vi "TL27_Display_Fault_Snapshot_Data_Parser rev4.vi"(5 "Input Snao Data":T3) -> (6 "Output Snap Data":T2[](array[typedef]))   [LabVIEW 2016]
uses:
  Get Raw Fault Snapshot Data.ctl
  Control 6.ctl
panel:
  in  "Parser Output Bundle 2":T1
  out "Boolean array":bool[](array[boolean])
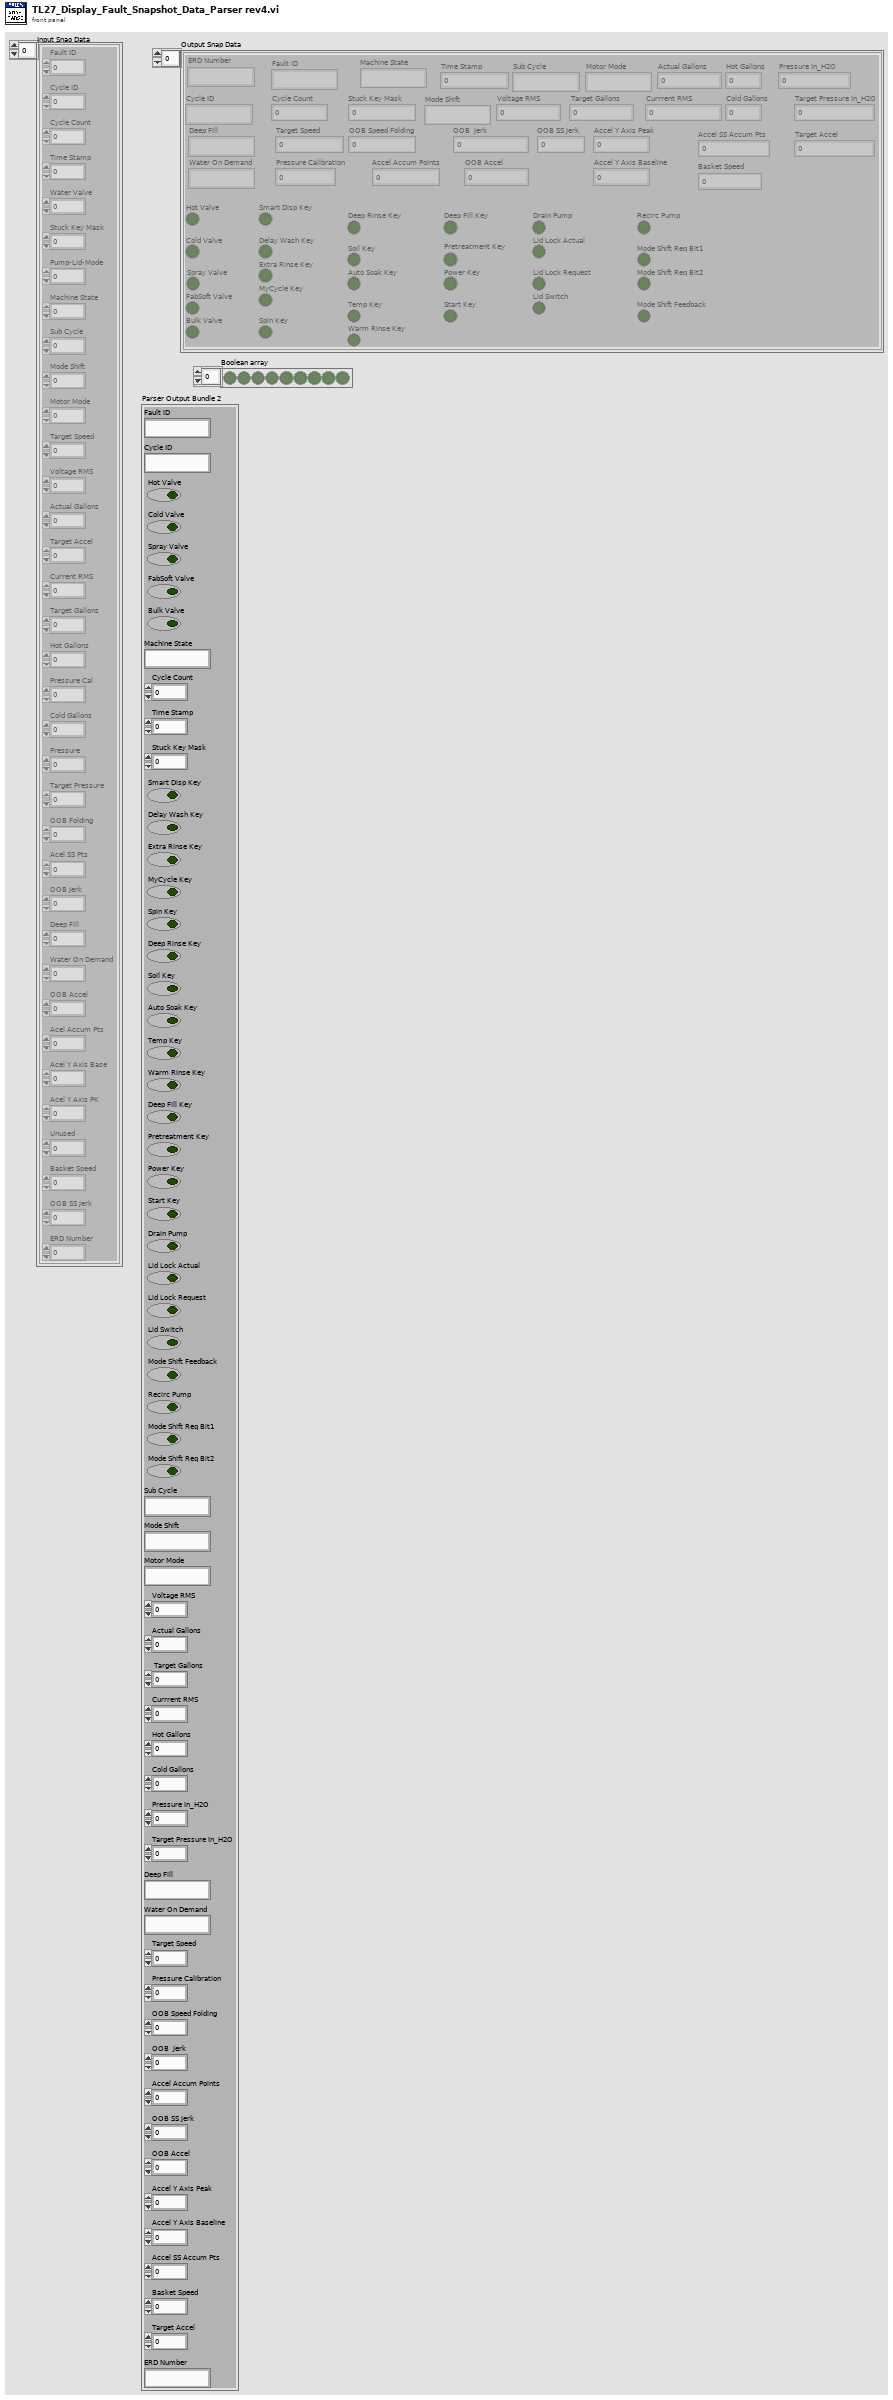
[diagram p1: front panel]
types:
  T1 = cluster{"Fault ID":string, "Cycle ID":string, "Hot Valve":bool, "Cold Valve":bool, "Spray Valve":bool, "FabSoft Valve":bool, "Bulk Valve":bool, "Machine State":string, "Cycle Count":u32, "Time Stamp":u32, "Stuck Key Mask ":u64, "Smart Disp Key":bool, "Delay Wash Key":bool, "Extra Rinse Key":bool, "MyCycle Key":bool, "Spin Key":bool, "Deep Rinse Key":bool, "Soil Key":bool, "Auto Soak Key":bool, "Temp Key":bool, "Warm Rinse Key":bool, "Deep Fill Key":bool, "Pretreatment Key":bool, "Power Key":bool, "Start Key":bool, "Drain Pump":bool, "Lid Lock Actual":bool, "Lid Lock Request":bool, "Lid Switch":bool, "Mode Shift Feedback":bool, "Recirc Pump":bool, "Mode Shift Req Bit1":bool, "Mode Shift Req Bit2":bool, "Sub Cycle":string, "Mode Shift":string, "Motor Mode":string, "Voltage RMS":u16, "Actual Gallons":u16, " Target Gallons":u16, "Currrent RMS":u16, "Hot Gallons":u16, "Cold Gallons":u16, "Pressure In_H2O":u32, "Target Pressure In_H2O":dbl, "Deep Fill":string, "Water On Demand":string, "Target Speed":u16, "Pressure Calibration":u32, "OOB Speed Folding":i32, "OOB  Jerk":i32, "Accel Accum Points":u8, "OOB SS Jerk":i32, "OOB Accel":i32, "Accel Y Axis Peak":i16, "Accel Y Axis Baseline":i16, "Accel SS Accum Pts":u8, "Basket Speed":u16, "Target Accel":u16, "ERD Number":string}
  T2 = typedef "Control 6.ctl" = cluster{"Fault ID":string, "Cycle ID":string, "Hot Valve":bool, "Cold Valve":bool, "Spray Valve":bool, "FabSoft Valve":bool, "Bulk Valve":bool, "Machine State":string, "Cycle Count":u32, "Time Stamp":u32, "Stuck Key Mask ":u64, "Smart Disp Key":bool, "Delay Wash Key":bool, "Extra Rinse Key":bool, "MyCycle Key":bool, "Spin Key":bool, "Deep Rinse Key":bool, "Soil Key":bool, "Auto Soak Key":bool, "Temp Key":bool, "Warm Rinse Key":bool, "Deep Fill Key":bool, "Pretreatment Key":bool, "Power Key":bool, "Start Key":bool, "Drain Pump":bool, "Lid Lock Actual":bool, "Lid Lock Request":bool, "Lid Switch":bool, "Mode Shift Feedback":bool, "Recirc Pump":bool, "Mode Shift Req Bit1":bool, "Mode Shift Req Bit2":bool, "Sub Cycle":string, "Mode Shift":string, "Motor Mode":string, "Voltage RMS":u16, "Actual Gallons":u16, " Target Gallons":u16, "Currrent RMS":u16, "Hot Gallons":u16, "Cold Gallons":u16, "Pressure In_H2O":u32, "Target Pressure In_H2O":dbl, "Deep Fill":string, "Water On Demand":string, "Target Speed":i16, "Pressure Calibration":u32, "OOB Speed Folding":i32, "OOB  Jerk":i32, "Accel Accum Points":u8, "OOB SS Jerk":i32, "OOB Accel":i32, "Accel Y Axis Peak":i16, "Accel Y Axis Baseline":i16, "Accel SS Accum Pts":u8, "Basket Speed":u16, "Target Accel":u16, "ERD Number":string}
  T3 = typedef "Get Raw Fault Snapshot Data.ctl" = cluster{"Fault ID":u16, "Cycle ID":u8, "Cycle Count":u32, "Time Stamp":u32, "Water Valve":u8, "Stuck Key Mask":u64, "Pump-Lid-Mode":u8, "Machine State":u8, "Sub Cycle":u8, "Mode Shift":u8, "Motor Mode":u8, "Target Speed":i16, "Voltage RMS":u16, "Actual Gallons":u16, "Target Accel":u16, "Current RMS":u16, "Target Gallons":u16, "Hot Gallons":u16, "Pressure Cal":u32, "Cold Gallons":u16, "Pressure ":u32, "Target Pressure":u32, "OOB Folding":i32, "Acel SS Pts":u8, "OOB Jerk":i32, "Deep Fill":u8, "Water On Demand":u8, "OOB Accel":i32, "Acel Accum Pts":u8, "Acel Y Axis Base":i16, "Acel Y Axis PK":i16, "Unused":u8, "Basket Speed":u16, "OOB SS Jerk":i32, "ERD Number":u64}[]
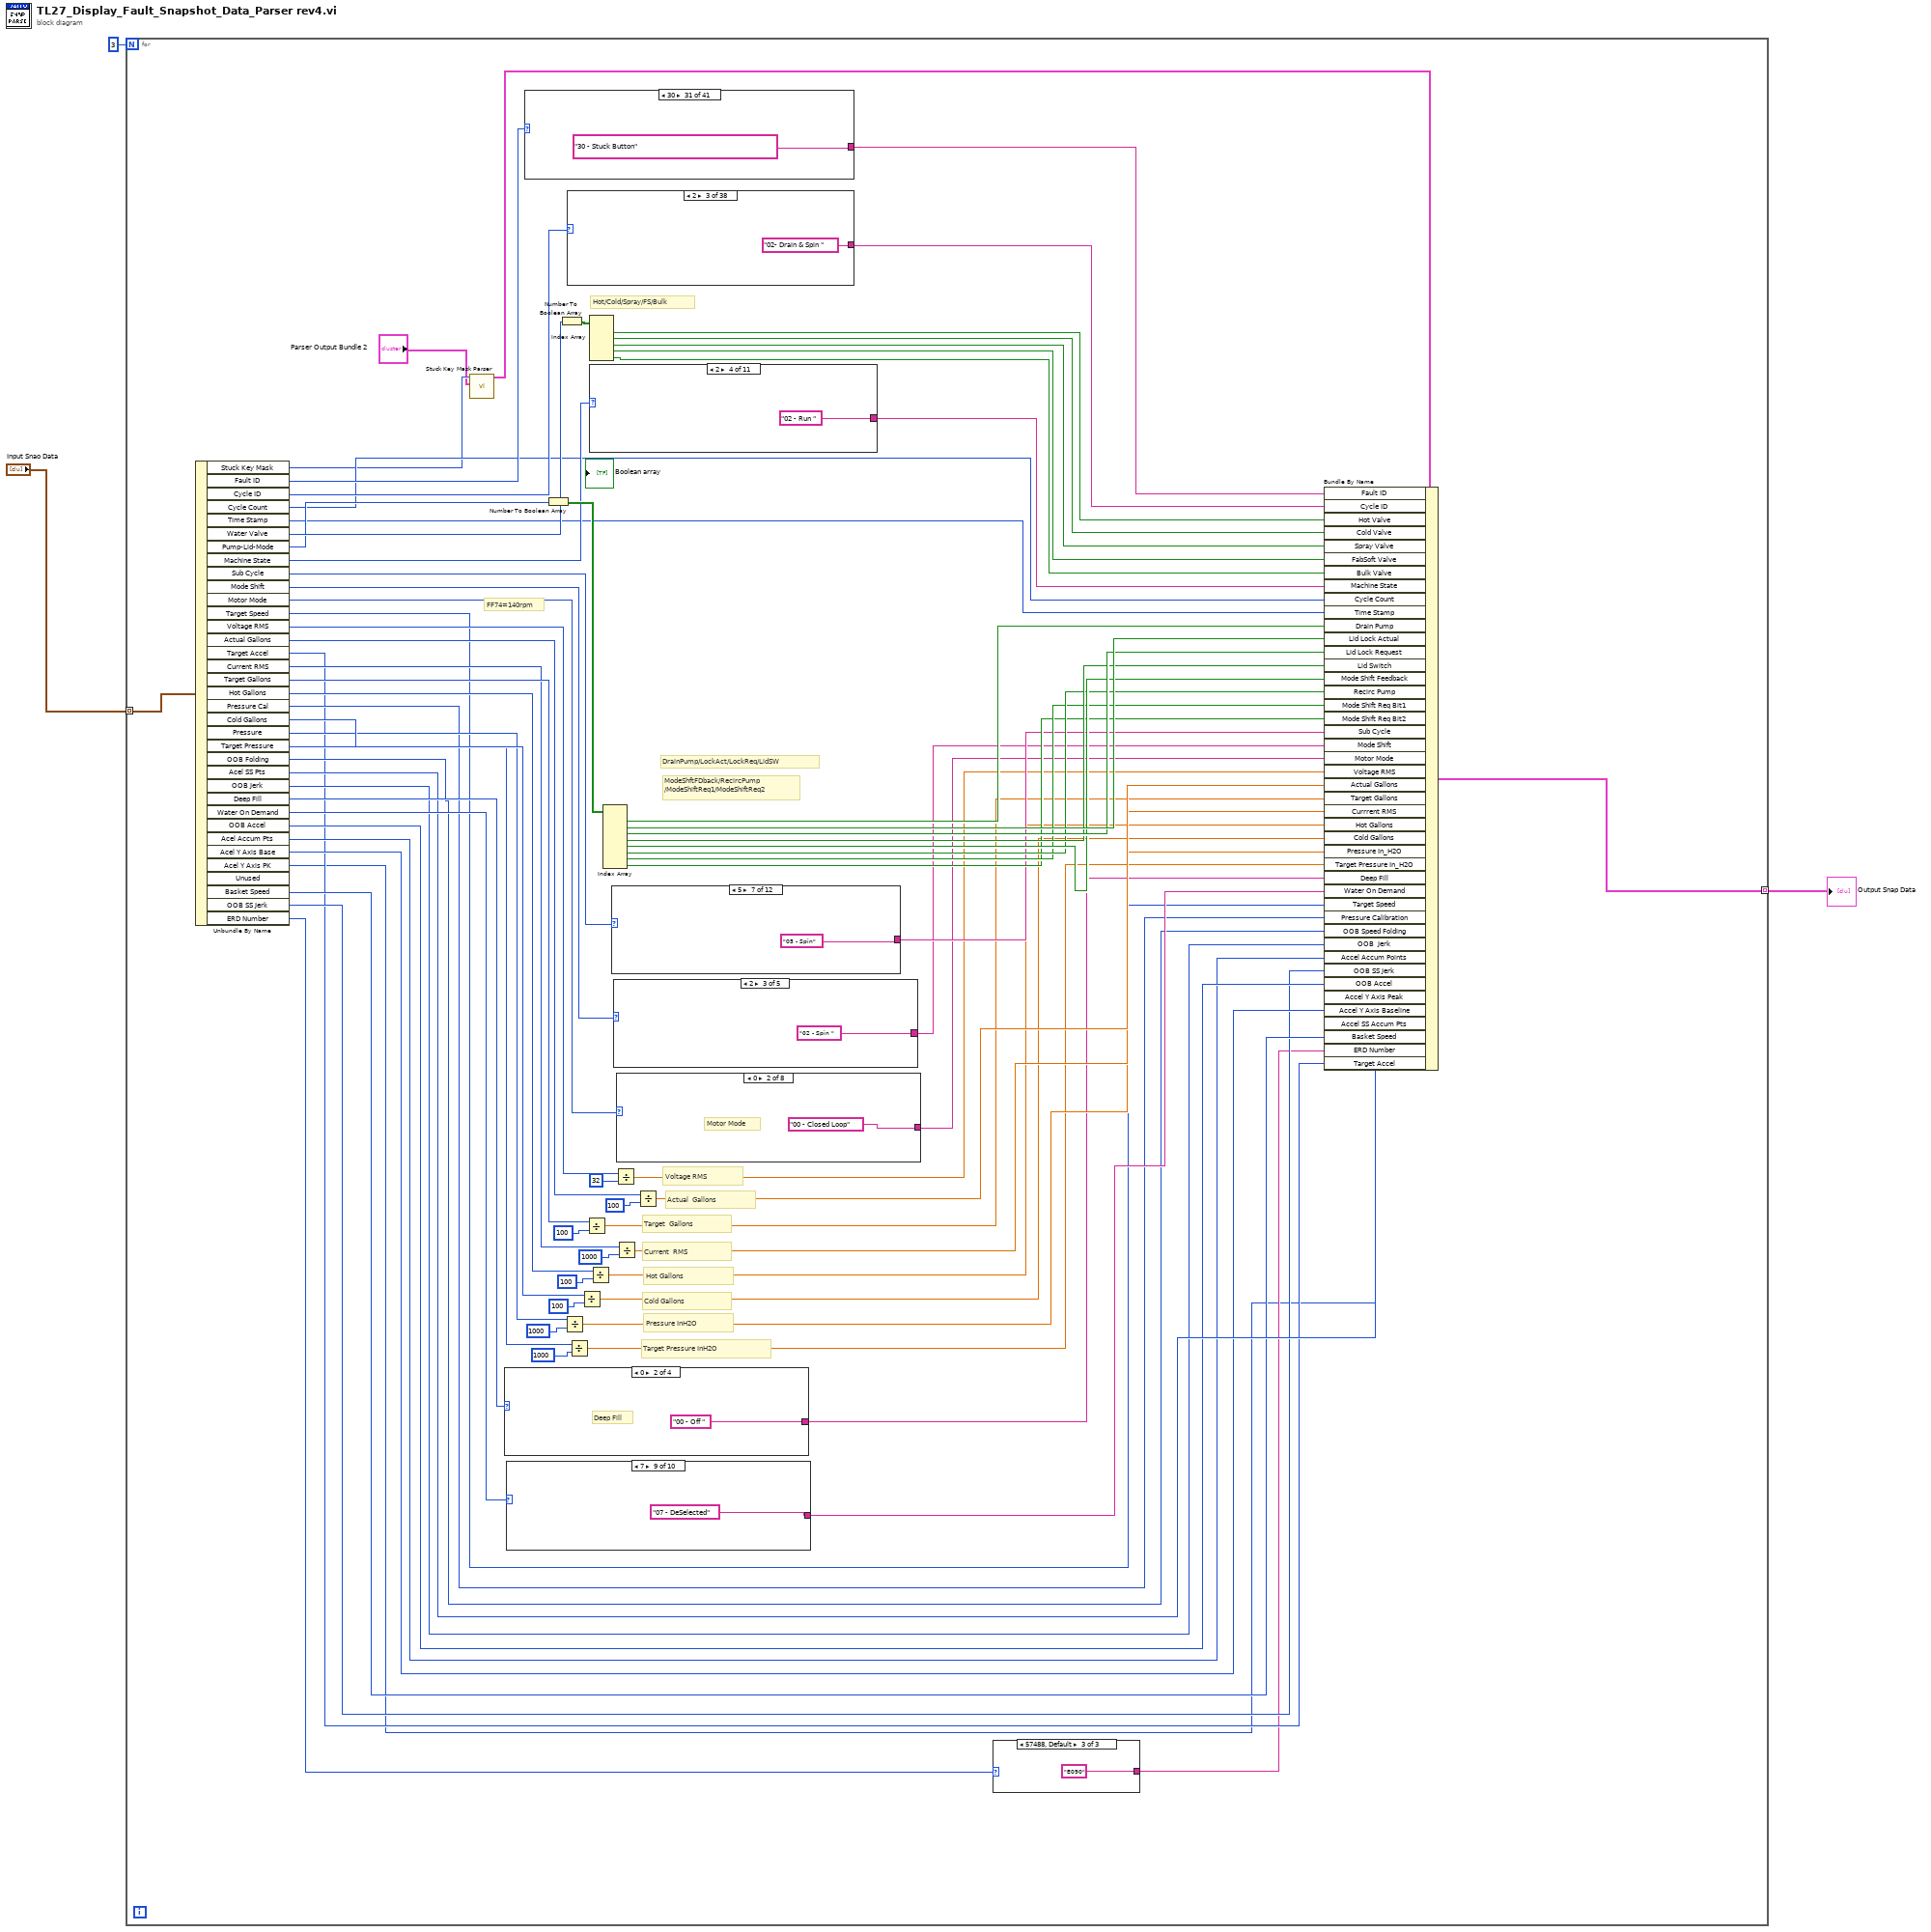
[diagram p0: block diagram]
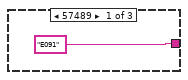
[diagram p2: hidden frame]
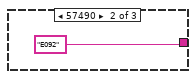
[diagram p3: hidden frame]
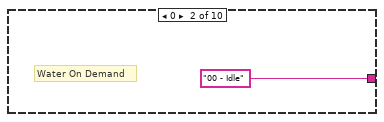
[diagram p5: hidden frame]
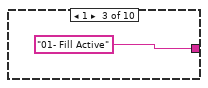
[diagram p6: hidden frame]
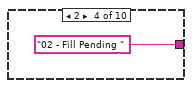
[diagram p7: hidden frame]
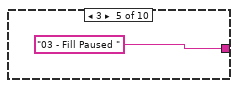
[diagram p8: hidden frame]
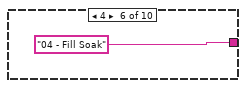
[diagram p9: hidden frame]
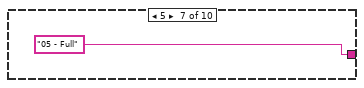
[diagram p10: hidden frame]
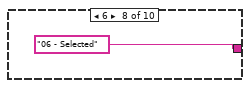
[diagram p11: hidden frame]
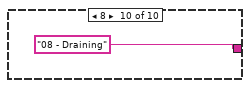
[diagram p12: hidden frame]
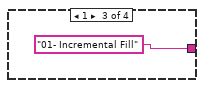
[diagram p14: hidden frame]
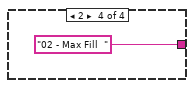
[diagram p15: hidden frame]
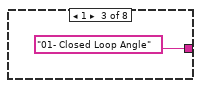
[diagram p17: hidden frame]
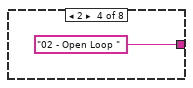
[diagram p18: hidden frame]
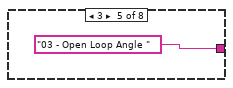
[diagram p19: hidden frame]
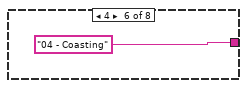
[diagram p20: hidden frame]
diagram:
  n1 = for {
    N: 3 -> [_]
    tunnel: "Input Snao Data" -> [w81] mode=indexing
    tunnel: [w10] -> w1 mode=indexing
    # "Target Pressure InH2O"
    # "Pressure InH2O"
    # "Cold Gallons"
    # "Hot Gallons"
    # "Current  RMS"
    # "Target  Gallons"
    # "Actual  Gallons"
    # "Voltage RMS"
    # "FF74=140rpm"
    # "ModeShftFDback/RecircPump\n/ModeShiftReq1/ModeShiftReq2"
    # "DrainPump/LockAct/LockReq/LidSW"
    # "Hot/Cold/Spray/FS/Bulk"
    n2 = Unbundle By Name(w81) -> ("Stuck Key Mask"=w6:u64, "Fault ID"=w80:u16, "Cycle ID"=w79:u8, "Cycle Count"=w46:u32, "Time Stamp"=w45:u32, "Water Valve"=w77:u8, "Pump-Lid-Mode"=w76:u8, "Machine State"=w74:u8, "Sub Cycle"=w73:u8, "Mode Shift"=w72:u8, "Motor Mode"=w71:u8, "Target Speed"=w8:i16, "Voltage RMS"=w70:u16, "Actual Gallons"=w67:u16, "Target Accel"=w13:u16, "Current RMS"=w63:u16, "Target Gallons"=w65:u16, "Hot Gallons"=w61:u16, "Pressure Cal"=w22:u32, "Cold Gallons"=w59:u16, "Pressure"=w57:u32, "Target Pressure"=w56:u32, "OOB Folding"=w21:i32, "Acel SS Pts"=w20:u8, "OOB Jerk"=w19:i32, "Deep Fill"=w55:u8, "Water On Demand"=w54:u8, "OOB Accel"=w18:i32, "Acel Accum Pts"=w17:u8, "Acel Y Axis Base"=w16:i16, "Acel Y Axis PK"=w9:i16, "Basket Speed"=w15:u16, "OOB SS Jerk"=w14:i32, "ERD Number"=w11:u64)  [unwired: 1 out]
    n3 = call "Stuck Key Mask Parser.vi"("Parser Output Bundle"="Parser Output Bundle 2", "Stuck Key Mask"=w6) -> ("output cluster"=w5:T1)  [unwired: 8 in, 1 out]
    n4 = case shown="0" w55 {
      tunnel: [_ "00 - Off " "01- Incremental Fill" "02 - Max Fill  "] -> w24
      frame 3, Default {
      }
      frame 0 {
        # "Deep Fill"
      }
      frame 1 {
      }
      frame 2 {
      }
    }
    n5 = case shown="7" w54 {
      tunnel: [_ "00 - Idle" "01- Fill Active" "02 - Fill Pending " "03 - Fill Paused " "04 - Fill Soak" "05 - Full" "06 - Selected" "07 - DeSelected" "08 - Draining"] -> w23
      frame 9, Default {
      }
      frame 0 {
        # "Water On Demand"
      }
      frame 1 {
      }
      frame 2 {
      }
      frame 3 {
      }
      frame 4 {
      }
      frame 5 {
      }
      frame 6 {
      }
      frame 7 {
      }
      frame 8 {
      }
    }
    n6 = case shown="30" w80 {
      tunnel: ["No Fault" "01- Lock Monitor" "02- Lid Monitor " "03 - Locked Rotor " "04 - Unused" "05 - Mode Shift" "06 - Critical Flood Level by Pressure" "07 - Unused" "08 - Pressure Sensor Loss" "09 - Lid Switch Redundancy" "10 - Mode Shift Feedback Monitor" "11 - Unused" "12 - Redundant Flood" "13 - Redundant Lid Unlocked" "14 - Unused" "15 - Temp Sensor Invalid" "16 - Unused" "17 - Dry Load Sense Timeout" "18 - Drain Pump Clearing" "19 - UI State Timeout" "20 - Critical Flood Level by Gallons" "21 - Unused" "22 - OOB During Dry Load Sense" "23 - Critical Lid Lock: Can't Lock" "24 - Lid Logic Failure" "25 - Pressure Sensor Dropout" "26 - OOB Redistribution" "27 - Water Accessibility" "28 - ADC Knob Feedback Invalid" "29 - Suds Lock Abatement" "30 - Stuck Button" "31 - OOB Fallback In Final Spin" "32 - Critical Lid Lock: Can't Unlock" "100 - Accelerometer Comm Error" "101 - Max Fill Pressure" "102 - Clock Monitor " "103 = Lid Lock Failure" "104 - Adaptive Drain" "105 - Max Fill Volume" "106 - Target Spin Speed Timeout" "107 - Target Spin Speed Dropout"] -> w7
      frame 0, Default {
        # "Fault ID"
      }
      frame 1 {
      }
      frame 2 {
      }
      frame 3 {
      }
      frame 4 {
      }
      frame 5 {
      }
      frame 6 {
      }
      frame 7 {
      }
      frame 8 {
      }
      frame 9 {
      }
      frame 10 {
      }
      frame 11 {
      }
      frame 12 {
      }
      frame 13 {
      }
      frame 14 {
      }
      frame 15 {
      }
      frame 16 {
      }
      frame 17 {
      }
      frame 18 {
      }
      frame 19 {
      }
      frame 20 {
      }
      frame 21 {
      }
      frame 22 {
      }
      frame 23 {
      }
      frame 24 {
      }
      frame 25 {
      }
      frame 26 {
      }
      frame 27 {
      }
      frame 28 {
      }
      frame 29 {
      }
      frame 30 {
      }
      frame 31 {
      }
      frame 32 {
      }
      frame 100 {
      }
      frame 101 {
      }
      frame 102 {
      }
      frame 103 {
      }
      frame 104 {
      }
      frame 105 {
      }
      frame 106 {
      }
      frame 107 {
      }
    }
    n7 = Number To Boolean Array(number=w76) -> (Boolean array=w75:bool[])
    n8 = Number To Boolean Array(number=w77) -> (Boolean array=w78:bool[])
    n9 = Divide(x=w57, y=u16 1000) -> (x/y=w27:dbl)
    n10 = case shown="2" w79 {
      tunnel: ["Not Defined" "01- Basket Clean" "02- Drain & Spin " "03 - Quick Rinse " "04 - Bulky Items" "05 - Sanitize" "06 - Towels / Sheets" "08 - Normal Mixed Load" "09 - Whites" "10 - Dark Colors" "11 - Jeans" "12 - Hand Wash" "13 - Delicates" "14 - Speed Wash" "15 - Heavy Duty" "16 - Allergen" "17 - Power Clean" "18 - Rinse & Spin" "19 - Single Item Wash" "20 - Colors" "21 - Cold Wash" "22 - Not Used-Start" "127 - Not Used-End" "128 - Cottons" "129 - Easy Care " "130 - Active Wear" "131 - Timed Dry" "132 - DeWrinkle" "133 - Quick Air Fluff" "134 - Steam Refresh" "135 - Steam DeWrinkle" "136 - Speed Dry" "137 - Mixed" "138 - Quick Dry" "139 - Casuals" "140 - WarmUp" "141 - Energy Saver" "142 - Antibacterial"] -> w53
      frame 0, Default {
        # "Cycle ID"
      }
      frame 1 {
      }
      frame 2 {
      }
      frame 3 {
      }
      frame 4 {
      }
      frame 5 {
      }
      frame 6 {
      }
      frame 8 {
      }
      frame 9 {
      }
      frame 10 {
      }
      frame 11 {
      }
      frame 12 {
      }
      frame 13 {
      }
      frame 14 {
      }
      frame 15 {
      }
      frame 16 {
      }
      frame 17 {
      }
      frame 18 {
      }
      frame 19 {
      }
      frame 20 {
      }
      frame 21 {
      }
      frame 22 {
      }
      frame 127 {
      }
      frame 128 {
      }
      frame 129 {
      }
      frame 130 {
      }
      frame 131 {
      }
      frame 132 {
      }
      frame 133 {
      }
      frame 134 {
      }
      frame 135 {
      }
      frame 136 {
      }
      frame 137 {
      }
      frame 138 {
      }
      frame 139 {
      }
      frame 140 {
      }
      frame 141 {
      }
      frame 142 {
      }
    }
    n11 = Divide(x=w56, y=u16 1000) -> (x/y=w25:dbl)
    n12 = Divide(x=w59, y=u16 100) -> (x/y=w28:dbl)
    n13 = Divide(x=w65, y=u16 100) -> (x/y=w31:dbl)
    n14 = Divide(x=w61, y=u16 100) -> (x/y=w29:dbl)
    n15 = Index Array(array=w78) -> (element #1=w52:bool, element #2=w51:bool, element #3=w50:bool, element #4=w49:bool, element #5=w48:bool)  [unwired: 5 in]
    n16 = case shown="2" w74 {
      tunnel: [_ "00 - Idle" "01- Standby" "02 - Run " "03 - Pause " "04 - EOC" "05 - DSMDelayRun" "06 - Delay Run" "07 - Delay Pause" "08 - Drain Timeout" "128 - Clean Speak"] -> w47
      frame 9, Default {
      }
      frame 0 {
        # "Machine State"
      }
      frame 1 {
      }
      frame 2 {
      }
      frame 3 {
      }
      frame 4 {
      }
      frame 5 {
      }
      frame 6 {
      }
      frame 7 {
      }
      frame 8 {
      }
      frame 128 {
      }
    }
    n17 = Index Array(array=w75) -> (element #1=w44:bool, element #2=w43:bool, element #3=w42:bool, element #4=w41:bool, element #5=w40:bool, element #6=w39:bool, element #7=w38:bool, element #8=w37:bool)  [unwired: 8 in]
    n18 = case shown="5" w73 {
      tunnel: [_ "00 - Not Applicable" "01- Fill" "02 - Soak " "03 - Wash " "04 - Rinse" "05 - Spin" "06 - Drain" "07 - Extra Spin" "08 - Extra Rinse" "128 - Tumble" "10 - Load Size Detection"] -> w36
      frame 11, Default {
      }
      frame 0 {
        # "Sub Cycle"
      }
      frame 1 {
      }
      frame 2 {
      }
      frame 3 {
      }
      frame 4 {
      }
      frame 5 {
      }
      frame 6 {
      }
      frame 7 {
      }
      frame 8 {
      }
      frame 9 {
      }
      frame 10 {
      }
    }
    n19 = case shown="2" w72 {
      tunnel: ["00 - Unknown" "01- Agitate" "02 - Spin " "03 - Transition to Spin " "04 - Transition to Agitate"] -> w35
      frame 0, Default {
        # "Mode Shift"
      }
      frame 1 {
      }
      frame 2 {
      }
      frame 3 {
      }
      frame 4 {
      }
    }
    n20 = Divide(x=w70, y=u16 32) -> (x/y=w33:dbl)
    n21 = Divide(x=w63, y=u16 1000) -> (x/y=w30:dbl)
    n22 = case shown="0" w71 {
      tunnel: [_ "00 - Closed Loop" "01- Closed Loop Angle" "02 - Open Loop " "03 - Open Loop Angle " "04 - Coasting" "05 - Braking" "06 - Idle"] -> w34
      frame 7, Default {
      }
      frame 0 {
        # "Motor Mode"
      }
      frame 1 {
      }
      frame 2 {
      }
      frame 3 {
      }
      frame 4 {
      }
      frame 5 {
      }
      frame 6 {
      }
    }
    n23 = Divide(x=w67, y=u16 100) -> (x/y=w32:dbl)
    n24 = case shown="57488, Default" w11 {
      tunnel: ["E091" "E092" "E090"] -> w12
      frame 57489 {
      }
      frame 57490 {
      }
      frame 57488, Default {
      }
    }
    n25 = Bundle By Name(cluster=w5, "Fault ID"=w7, "Cycle ID"=w53, "Hot Valve"=w52, "Cold Valve"=w51, "Spray Valve"=w50, "FabSoft Valve"=w49, "Bulk Valve"=w48, "Machine State"=w47, "Cycle Count"=w46, "Time Stamp"=w45, "Drain Pump"=w44, "Lid Lock Actual"=w43, "Lid Lock Request"=w42, "Lid Switch"=w41, "Mode Shift Feedback"=w40, "Recirc Pump"=w39, "Mode Shift Req Bit1"=w38, "Mode Shift Req Bit2"=w37, "Sub Cycle"=w36, "Mode Shift"=w35, "Motor Mode"=w34, "Voltage RMS"=w33, "Actual Gallons"=w32, "Target Gallons"=w31, "Currrent RMS"=w30, "Hot Gallons"=w29, "Cold Gallons"=w28, "Pressure In_H2O"=w27, "Target Pressure In_H2O"=w25, "Deep Fill"=w24, "Water On Demand"=w23, "Target Speed"=w8, "Pressure Calibration"=w22, "OOB Speed Folding"=w21, "OOB  Jerk"=w19, "Accel Accum Points"=w17, "OOB SS Jerk"=w14, "OOB Accel"=w18, "Accel Y Axis Peak"=w9, "Accel Y Axis Baseline"=w16, "Accel SS Accum Pts"=w20, "Basket Speed"=w15, "ERD Number"=w12, "Target Accel"=w13) -> (w10:T1)
  }
  "Output Snap Data" <- w1
